vi "Disconnect.vi"(8 "error in (no error)":errorcluster, 11 "Network Stream Writer in":refnum<class "Network Stream Writer.lvclass">) -> (0 "error out":errorcluster, 3 "Network Stream Writer out":refnum<class "Network Stream Writer.lvclass">)   [LabVIEW 2014, in "Network Stream Writer.lvlib" / "Network Stream Writer.lvclass"]
uses:
  Network Stream Writer.lvclass
  <vilib>/dex/Flush And Wait Empty Condition.ctl
  Network Stream/Network Stream/MessageString.ctl
  <vilib>/ActorFramework/Message Enqueuer/Message Priority.ctl
  Network Stream Writer.lvclass/Network Stream Writer.ctl
  Proxy/Proxy/Proxy.lvclass/Proxy.ctl
  <vilib>/ActorFramework/Actor/Actor.lvclass/Actor.ctl
  Proxy/Proxy Messages/Proxy Status Msg/Proxy Status Msg.lvclass/Proxy Status Msg.ctl
  Proxy/Proxy/Read Target Enq.vi
  Proxy/Proxy/Read Status Msg.vi
  <vilib>/ActorFramework/Message Enqueuer/Equals Not A Refnum.vi
  <vilib>/ActorFramework/Actor/Read Caller Enqueuer.vi
  <vilib>/ActorFramework/Message Enqueuer/Message Enqueuer.lvclass
  Proxy/Proxy Messages/Proxy Status Msg/Proxy Status Msg.lvclass
  Network Stream/Network Stream/Network Stream.lvclass
  <resource>/objmgr/ni.dex.rc
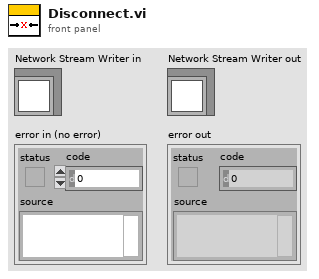
[diagram p1: front panel]
types:
  T1 = typedef "Flush And Wait Empty Condition.ctl" = u8
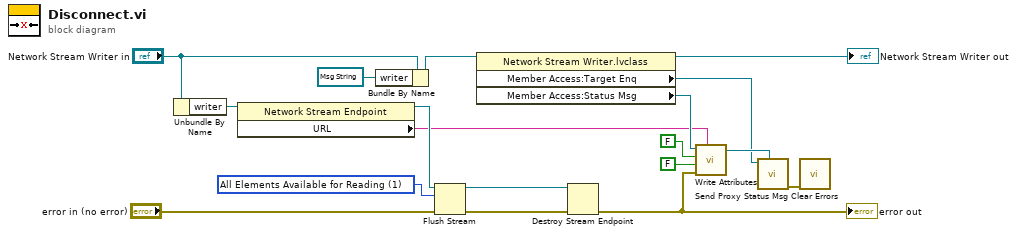
[diagram p0: block diagram]
diagram:
  w18 = T1 1 items=["All Elements Read From Stream", "All Elements Available for Reading"] ("wait condition")
  n1 = Unbundle By Name("Network Stream Writer in") -> ("writer"=w15:refnum<k21>)
  n2 = property class="Network Stream Endpoint"(reference=w15) -> (reference out=w4:refnum<k21>, "URL"=w3:string)  [unwired: 1 in, 1 out]
  n3 = Bundle By Name(cluster="Network Stream Writer in", "writer"=refnum<k21> refnum) -> (w12:refnum<class "Network Stream Writer.lvclass">)
  n4 = Flush Stream(8:"error in (no error)", 10:w18, 11:w4) -> (0:w16:errorcluster, 3:w17:refnum<k21>)  [unwired: 1 in, 1 out]
  n5 = property class="Network Stream Writer.lvclass"(reference=w12) -> (reference out=→"Network Stream Writer out":refnum<class "Network Stream Writer.lvclass">, "Member Access:Target Enq"=w8:refnum<class "Message Enqueuer.lvclass">, "Member Access:Status Msg"=w5:refnum<class "Proxy Status Msg.lvclass">)  [unwired: 1 in, 1 out]
  n6 = Destroy Stream Endpoint(8:w16, 11:w17) -> (0:w7:errorcluster)
  "error out" <- w7
  n7 = call "Write Attributes.vi"("Name"=w3, "error in"=w7, "Reader"=FALSE, "Writer"=FALSE, "Proxy Status Msg in"=w5) -> ("Proxy Status Msg out"=w10:refnum<class "Proxy Status Msg.lvclass">)  [unwired: 6 in]
  n8 = call "Send Proxy Status Msg.vi"("Message Type"=w10, "Message Enqueuer"=w8) -> ("error out"=w6:errorcluster)  [unwired: 8 in, 1 out]
  n9 = call <vilib>:"Clear Errors.vi"("error in (no error)"=w6) -> ()  [unwired: 5 in, 2 out]
